vi "GetContainerNames.vi"(8 "error in (no error)":errorcluster, 11 "CLabVIEWItem in":refnum<class "CLabVIEWItem.lvclass">) -> (0 "error out":errorcluster, 1 "Container name[]":string[](array[string]), 3 "CLabVIEWItem out":refnum<class "CLabVIEWItem.lvclass">)   [LabVIEW 2020, in "LabVIEWItem.lvlib" / "CLabVIEWItem.lvclass"]
uses:
  CLabVIEWItem.lvclass
  CLabVIEWItem.lvclass/CLabVIEWItem.ctl
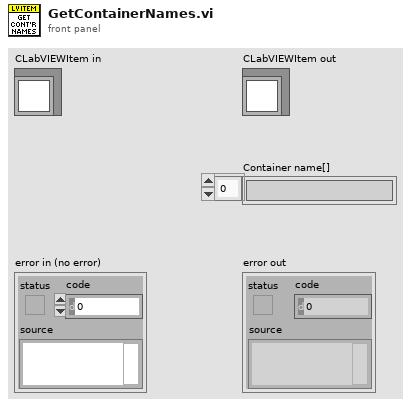
[diagram p1: front panel]
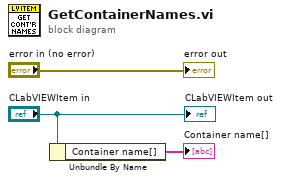
[diagram p0: block diagram]
diagram:
  n1 = Unbundle By Name("CLabVIEWItem in") -> ("Container name[]"=→"Container name[]":string[])
  "error out" <- "error in (no error)"
  "CLabVIEWItem out" <- "CLabVIEWItem in"
